vi "Server_right_joint_command.vi"() -> ()   [LabVIEW 2013]
doc: "Template server that runs individual ros topics, services, etc. This is cloned for each topic being run."
uses:
  ROS/Code/SubVIs/_ROSControl.ctl
  ROS/Code/SubVIs/_ROSDirection.ctl
  ROS/RosMessages/Clusters/JointCommand.ctl
panel:
  out "msg out (HEX)":string
  in  "New Port?":bool
  in  "JointCommand":T1={"Mode"=enum."Position", "Arm Angles"=[-0.5235987755982988, -0.8726646259971648, 0.0, 0.7853981633974483, 0.0, 1.6580627893946132, 0.0], "Angle Names"=["right_s0", "right_s1", "right_e0", "right_e1", "right_w0", "right_w1", "right_w2"]}
  in  "queue":string="/robot/limb/right/joint_commandQueue"
  out "Connected":bool
  out "Status":T2(ring) caption="Connected?"
  out "Specs":T4={"Server"="/robot/limb/right/joint_command", "Node"="/labview", "Server Port"=51179, "URI (Subsc)"="", "Direction"=enum."Publisher"}
  in  "stop":bool
  out "error out":errorcluster={"status"=TRUE, "code"=1, "source"="TCP Close Connection in _right_joint_command_Server.vi"}
  out "Connections":T5(array[cluster])
  in  "Baxter":T6={"topic port"=59814, "Node"="/labview", "topic"="/robot/limb/right/joint_command", "type"="baxter_msgs/JointCommand", "node port"=7000, "error "={"status"=FALSE, "code"=0, "source"=""}, "Direction"=enum."Publisher", "APIs"=[]}
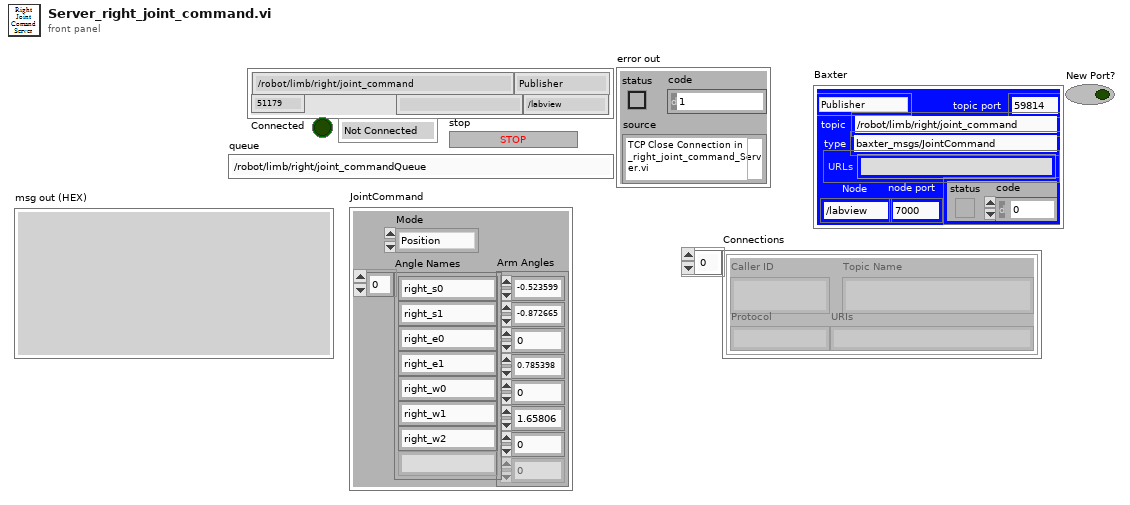
[diagram p1: front panel]
types:
  T1 = typedef "JointCommand.ctl" = cluster{"Mode":enum32{"", "Position", "Velocity", "Effort"}, "Arm Angles":dbl[], "Angle Names":string[]}
  T2 = enum16{"Not Connected", "Registered", "Connected"}
  T3 = typedef "_ROSDirection.ctl" = enum16{"Node", "Publisher", "Subscriber", "Service Client"}
  T4 = cluster{"Server":string, "Node":string, "Server Port":u32, "URI (Subsc)":string, "Direction":T3}
  T5 = cluster{"Caller ID":string, "Topic Name":string, "Protocol":string, "URIs":string}[]
  T6 = typedef "_ROSControl.ctl" = cluster{"topic port":u16, "Node":string, "topic":string, "type":string, "node port":u32, "error ":errorcluster, "Direction":T3, "APIs":string[]}
  T7 = cluster{"Caller ID":string, "Topic Name":string, "Protocol":string, "URIs":string}
  T8 = enum16{"big-endian, network order", "native, host order", "little-endian"}
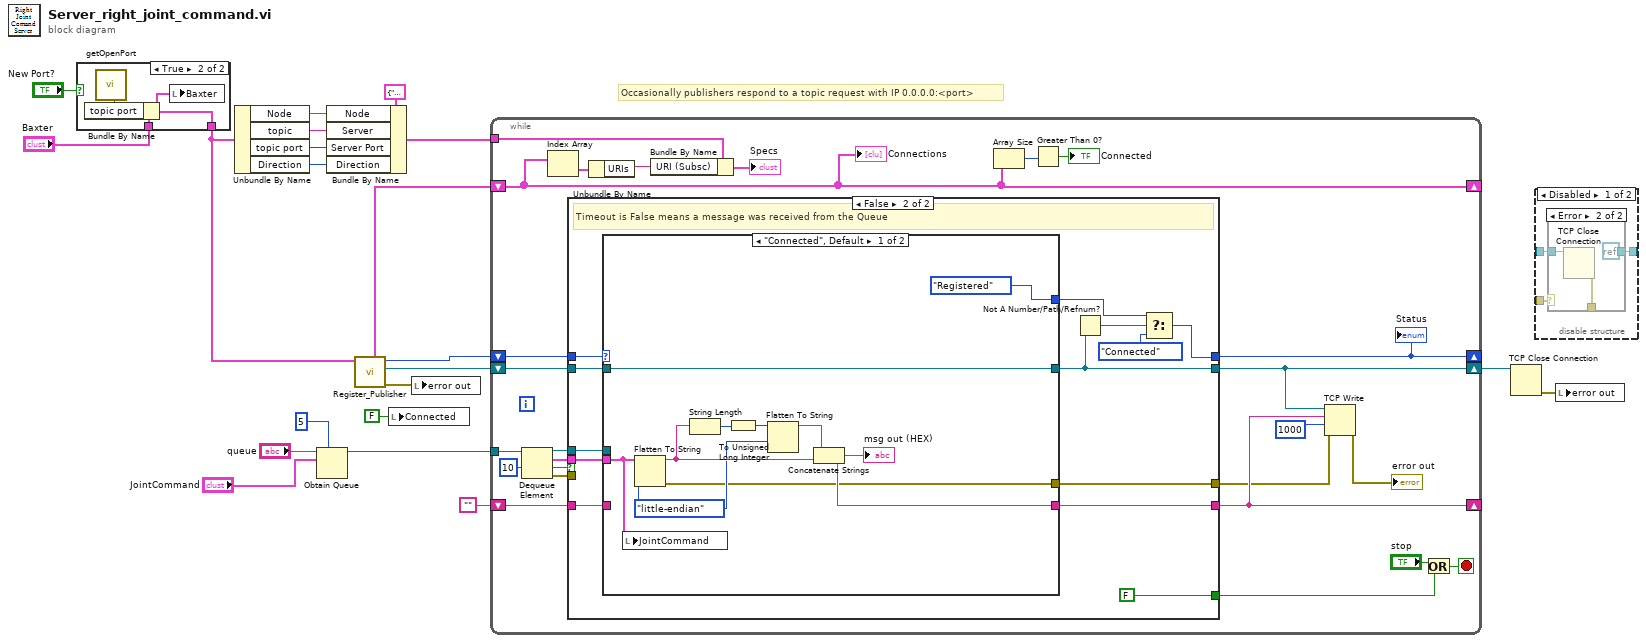
[diagram p0: block diagram]
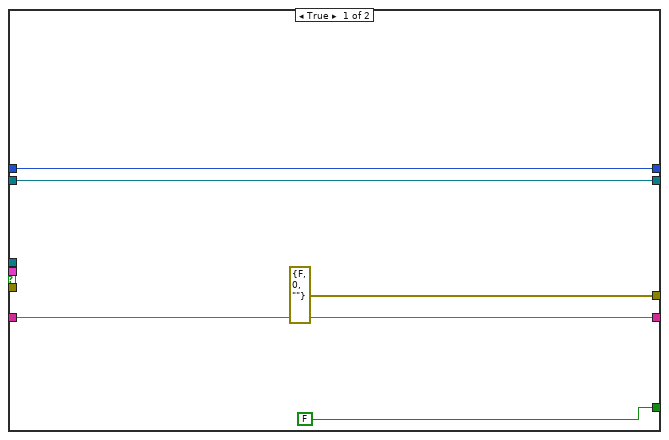
[diagram p5: hidden frame]
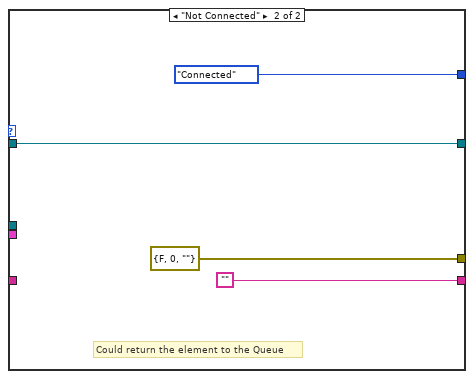
[diagram p6: hidden frame]
diagram:
  # "Occasionally publishers respond to a topic request with IP 0.0.0.0:<port>"
  n1 = case shown="True" "New Port?" {
    tunnel: "Baxter" -> [w22 w25]
    tunnel: [w22 w23] -> w8
    frame False {
    }
    frame True {
      n2 = call "getOpenPort.vi"() -> ("port"=w24:u16)
      n3 = Bundle By Name(cluster=w25, "topic port"=w24) -> (w23:T6)
      n4 = local write "Baxter"(w23) -> ()
    }
  }
  n5 = Unbundle By Name(w8) -> ("Node"=w19:string, "topic"=w18:string, "topic port"=w16:u16, "Direction"=w17:T3)
  n6 = Obtain Queue(max queue size (-1, unlimited)=5, name (unnamed)="queue", element data type="JointCommand") -> (queue out=w13:refnum<queue>)  [unwired: 2 in, 2 out]
  n7 = Bundle By Name(cluster=T4 {"Server"="", "Node"="/labview", "Server Port"=5000, "URI (Subsc)"="", "Direction"=enum."Node"} ("Specs"), "Node"=w19, "Server"=w18, "Server Port"=w16, "Direction"=w17) -> (w20:T4)
  n8 = call "Register_Publisher.vi"("Baxter"=w8) -> ("error out"=w5:errorcluster, "connection ID out"=w6:refnum<k5>, "Status"=w3:T2, "Subscribers"=w7:T5)  [unwired: 7 in]
  n9 = local write "Connected"(FALSE ("Connected")) -> ()
  n10 = local write "error out"(w5) -> ()
  n11 = while {
    shift-right: [w32] -> _
    shift-left: w7 -> [w32]
    shift-right: [w29] -> w12
    shift-left: w6 -> [w50]
    shift-right: [w47] -> _
    shift-left: w3 -> [w48]
    tunnel: w20 -> [w45]
    tunnel: w13 -> [w38]
    shift-right: [w28] -> _
    shift-left: "" -> [w31]
    stop <- w33 stop-if-true
    n12 = Dequeue Element(queue=w38, timeout in ms (-1)=10) -> (queue out=w42:refnum<queue>, element=w36:T1, timed out?=w37:bool, error out=w39:errorcluster)  [unwired: 1 in]
    n13 = Index Array(array=w32) -> (element=w46:T7)  [unwired: 1 in]
    n14 = case shown="False" w37 {
      tunnel: [w55 w65] -> w29
      tunnel: w50 -> [w55 w68]
      tunnel: [FALSE FALSE] -> w34
      tunnel: [errorcluster {"status"=FALSE, "code"=0, "source"=""} ("error out") w66] -> w27
      tunnel: w48 -> [w54 w67]
      tunnel: [w54 w60] -> w47
      tunnel: w42 -> [_ w64]
      tunnel: w39 -> [_ _]
      tunnel: w36 -> [_ w58]
      tunnel: [w51 w57] -> w28
      tunnel: w31 -> [w51 w56]
      frame True {
      }
      frame False {
        # "Timeout is False means a message was received from the Queue"
        n15 = case shown="\"Connected\", Default" w67 {
          tunnel: w68 -> [w70 w82]
          tunnel: [w70 w82] -> w65
          tunnel: [w69 errorcluster {"status"=FALSE, "code"=0, "source"=""} ("error out")] -> w66
          tunnel: w64 -> [_ _]
          tunnel: [T2."Registered" ("f") T2."Connected" ("f")] -> w61
          tunnel: w58 -> [w77 _]
          tunnel: [w71 ""] -> w57
          tunnel: w56 -> [_ _]
          frame "Connected", Default {
            w72 = T8."little-endian" ("byte order (0:big-endian, network order)")
            n16 = local write "JointCommand"(w77) -> ()
            n17 = Flatten To String(anything=w77, byte order (0:big-endian, network order)=w72) -> (data string=w73:string, error out=w69:errorcluster)  [unwired: 2 in, 1 out]
            n18 = String Length(string=w73) -> (length=w75:i32)
            n19 = To Unsigned Long Integer(number=w75) -> (unsigned 32bit integer=w74:u32)
            n20 = Flatten To String(anything=w74, byte order (0:big-endian, network order)=w72) -> (data string=w76:string)  [unwired: 2 in, 2 out]
            n21 = Concatenate Strings(w76, w73) -> (w71:string)
            "msg out (HEX)" <- w71
          }
          frame "Not Connected" {
            # "Could return the element to the Queue"
          }
        }
        n22 = Not A Number/Path/Refnum?(number/path/refnum=w65) -> (NaN/Path/Refnum?=w62:bool)
        n23 = Select(t=w61, s=w62, f=T2."Connected") -> (s? t:f=w60:T2)
      }
    }
    "Status" <- w47
    n24 = Unbundle By Name(w46) -> ("URIs"=w44:string)
    n25 = Bundle By Name(cluster=w45, "URI (Subsc)"=w44) -> (→"Specs":T4)
    n26 = Array Size(array=w32) -> (size(s)=w41:i32)
    n27 = Greater Than 0?(x=w41) -> (x > 0?=→"Connected":bool)
    n28 = TCP Write(connection ID=w29, data in=w28, error in (no error)=w27, 9:1000 ("timeout ms (25000)")) -> (error out=→"error out":errorcluster)  [unwired: 2 out]
    n29 = Or(x="stop", y=w34) -> (x .or. y?=w33:bool)
    "Connections" <- w32
  }
  n30 = TCP Close Connection(connection ID=w12) -> (error out=w11:errorcluster)  [unwired: 2 in, 1 out]
  n31 = disable-structure shown="Disabled" {
    disable-tunnel: _ -> [w85 _]
    disable-tunnel: [w84 _] -> _
    disable-tunnel: _ -> [w83 _]
    frame Disabled {
      n32 = case shown="Error" w85 {
        tunnel: w83 -> [w86 w89]
        tunnel: [w86 refnum<k0> refnum] -> w84
        tunnel: [_ w87] -> _
        frame No Error {
        }
        frame Error {
          n33 = TCP Close Connection(connection ID=w89) -> (error out=w87:errorcluster)  [unwired: 2 in, 1 out]
        }
      }
    }
    frame Enabled {
    }
  }
  n34 = local write "error out"(w11) -> ()
